vi "State Enter Core.vi"(8 "error in (no error)":errorcluster, 11 "B Context State in":refnum<class "B Context State.lvclass">) -> (0 "error out":errorcluster, 3 "B Context State out":refnum<class "B Context State.lvclass">)   [LabVIEW 2021, in "B Context State.lvclass"]
uses:
  B Context State.lvclass
  B Context State.lvclass/B Context State.ctl
  Context/Context.lvclass
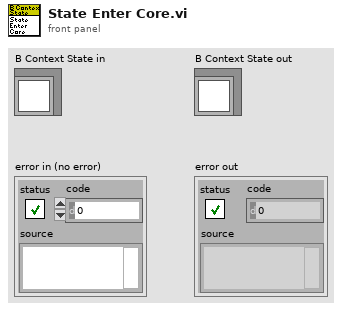
[diagram p1: front panel]
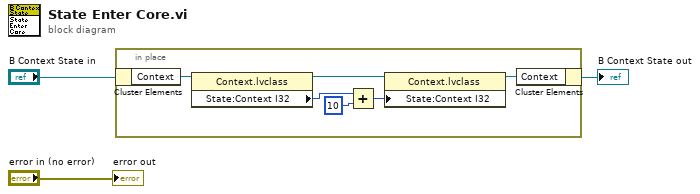
[diagram p0: block diagram]
diagram:
  n1 = in-place {
    n2 = in-place-cluster #1("B Context State in") -> ("Context"=w9:refnum<class "Context.lvclass">)
    n3 = property class="Context.lvclass"(reference=w9) -> (reference out=w8:refnum<class "Context.lvclass">, "State:Context I32"=w6:i32)  [unwired: 1 in, 1 out]
    n4 = Add(x=w6, y=10) -> (x+y=w5:i32)
    n5 = property class="Context.lvclass"(reference=w8, "State:Context I32"=w5) -> (reference out=w7:refnum<class "Context.lvclass">)  [unwired: 1 in, 1 out]
    n6 = in-place-cluster #1("Context"=w7) -> (→"B Context State out":refnum<class "B Context State.lvclass">)
  }
  "error out" <- "error in (no error)"
